vi "新增号数加1.vi"(2 "号数类型":enum16{"普通业务", "VIP业务", "其它业务"}(ring), 5 "原业务号":string) -> (1 "新增业务号":string)   [LabVIEW 2019]
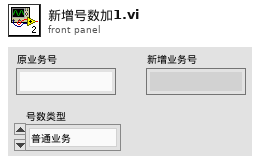
[diagram p1: front panel]
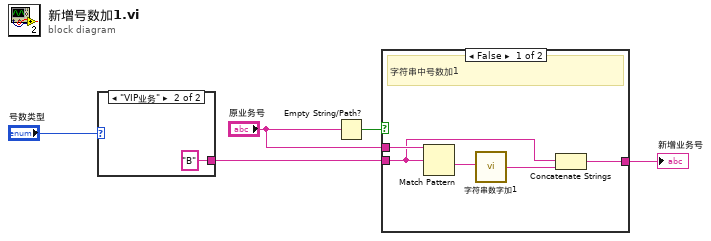
[diagram p0: block diagram]
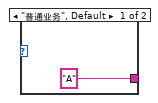
[diagram p2: hidden frame]
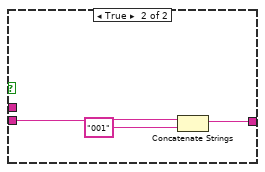
[diagram p3: hidden frame]
diagram:
  n1 = case shown="\"VIP业务\"" "号数类型" {
    tunnel: ["A" ("regular expression") "B" ("regular expression")] -> w1
    frame "普通业务", Default {
    }
    frame "VIP业务" {
    }
  }
  n2 = Empty String/Path?(string/path="原业务号") -> (empty?=w3:bool)
  n3 = case shown="False" w3 {
    tunnel: [w10 w13] -> w5
    tunnel: "原业务号" -> [w12 _]
    tunnel: w1 -> [w8 w15]
    frame False {
      # "字符串中号数加1"
      n4 = Match Pattern(string=w12, regular expression=w8) -> (after substring=w9:string)  [unwired: 1 in, 3 out]
      n5 = call "字符串数字加1.vi"("OldString"=w9) -> ("NewString"=w11:string)
      n6 = Concatenate Strings(w8, w11) -> (w10:string)
    }
    frame True {
      n7 = Concatenate Strings(w15, "001" ("新增VIP业务号")) -> (w13:string)
    }
  }
  "新增业务号" <- w5
